vi "Run Toolkit Unit Tests.vi"(8 "Error In":errorcluster) -> (0 "Error Out":errorcluster)   [LabVIEW 2018, in "Scripts.lvlib"]
uses:
  Scripts.lvlib
  Toolkit/Tests/Tests.lvlib
  <vilib>/addons/_JKI Toolkits/Caraya/classes/Test/Test.lvclass
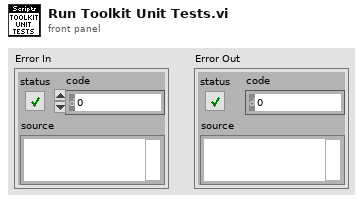
[diagram p1: front panel]
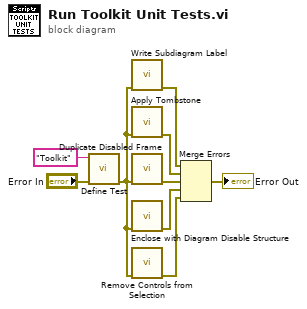
[diagram p0: block diagram]
diagram:
  n1 = call <vilib>:"Define Test.vi"("error in (no error)"="Error In", "Label (VI Title)"="Toolkit") -> ("error out"=w2:errorcluster)  [unwired: 9 in]
  n2 = call "Write Subdiagram Label.vi"("Error In"=w2) -> ("Error Out"=w3:errorcluster)  [unwired: 10 in]
  n3 = call "Apply Tombstone.vi"("Error In"=w2) -> ("Error Out"=w5:errorcluster)  [unwired: 10 in]
  n4 = call "Duplicate Disabled Frame.vi"("Error In"=w2) -> ("Error Out"=w6:errorcluster)  [unwired: 10 in]
  n5 = call "Enclose with Diagram Disable Structure.vi"("Error In"=w2) -> ("Error Out"=w7:errorcluster)  [unwired: 10 in]
  n6 = call "Remove Controls from Selection.vi"("Error In"=w2) -> ("Error Out"=w9:errorcluster)  [unwired: 10 in]
  n7 = Merge Errors(w3, w5, w6, w7, w9) -> (→"Error Out":errorcluster)
